vi "Calculate Radius (ball pick up).vi"() -> ()   [LabVIEW 2015]
uses:
  <vilib>/express/express arith-compare/Formula/XNode/ExpressFormulaBlockNode.xnode
panel:
  out "x = y?":bool
  out "Radius 2":dbl
  out "X of intersection":dbl
  out "Radius":dbl
  in  "math tolerance":dbl=0.06
  in  "Ball Y":dbl
  in  "Ball X":dbl
  in  "Min Detect Distance":dbl
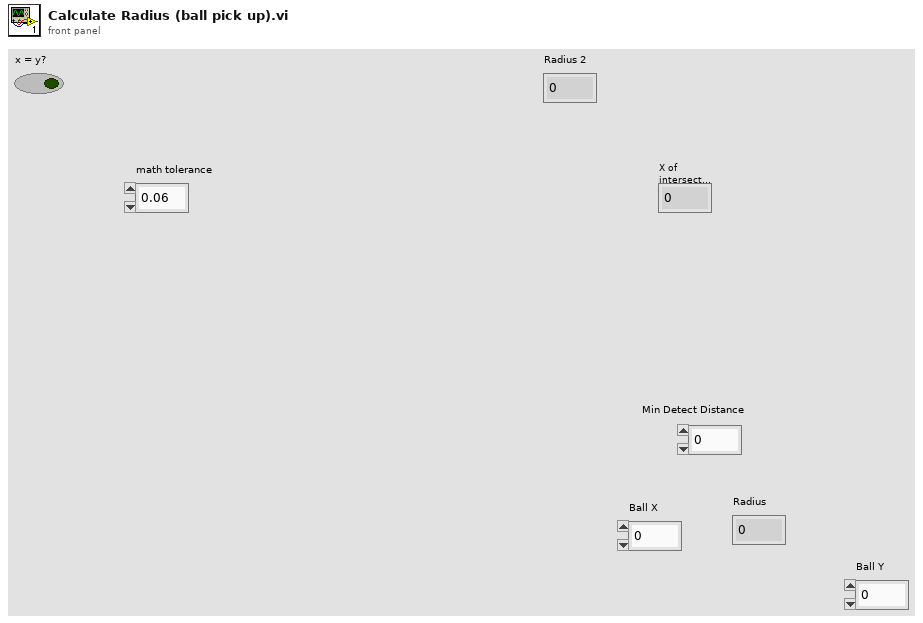
[diagram p1: front panel]
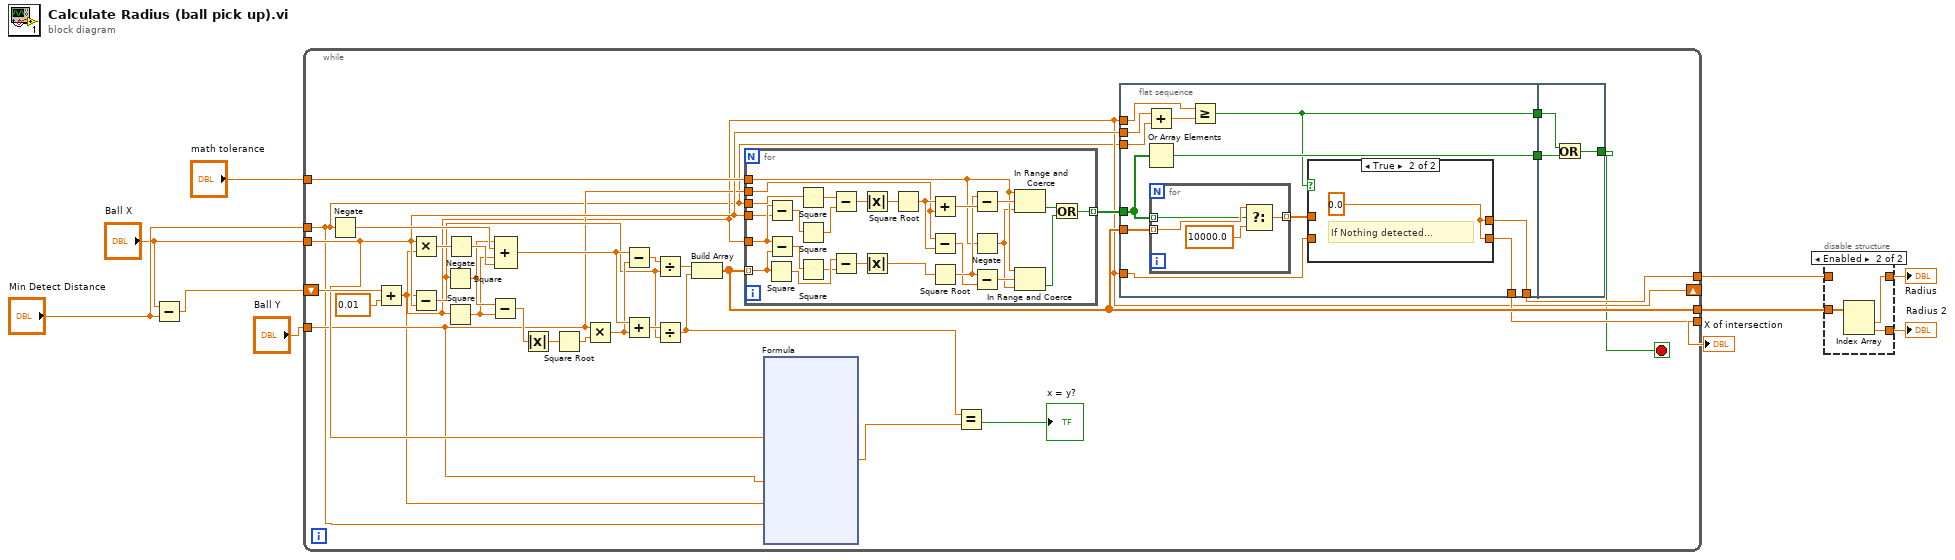
[diagram p0: block diagram]
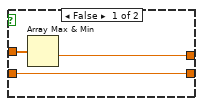
[diagram p3: hidden frame]
diagram:
  n1 = Subtract(x="Ball X", y="Min Detect Distance") -> (x-y=w8:dbl)
  n2 = while {
    tunnel: "Ball X" -> [w18]
    tunnel: "Min Detect Distance" -> [w15]
    shift-right: [w16] -> _
    shift-left: w8 -> [w41]
    tunnel: "Ball Y" -> [w17]
    tunnel: "math tolerance" -> [w26]
    tunnel: [w24] -> w3
    tunnel: [w19] -> w5
    tunnel: [w20] -> w2
    stop <- w11 stop-if-true
    n3 = Negate(x=w15) -> (-x=w39:dbl)
    n4 = Add(x=w41, y=0.01) -> (x+y=w16:dbl)
    n5 = Multiply(x=w18, y=w16) -> (x*y=w38:dbl)
    n6 = Subtract(x=w16, y=w18) -> (x-y=w28:dbl)
    n7 = Square(x=w28) -> (x^2=w35:dbl)
    n8 = Square(x=w16) -> (x^2=w34:dbl)
    n9 = Negate(x=w38) -> (-x=w37:dbl)
    n10 = Subtract(x=w35, y=w34) -> (x-y=w33:dbl)
    n11 = Compound Arithmetic op=ADD(w35, w39, w34, w37) -> (w31:dbl)
    n12 = Absolute Value(x=w33) -> (abs(x)=w21:dbl)
    n13 = Square Root(x=w21) -> (sqrt(x)=w36:dbl)
    n14 = Multiply(x=w17, y=w36) -> (x*y=w30:dbl)
    n15 = Subtract(x=w31, y=w30) -> (x-y=w29:dbl)
    n16 = Add(x=w31, y=w30) -> (x+y=w32:dbl)
    n17 = Divide(x=w29, y=w28) -> (x/y=w27:dbl)
    n18 = Divide(x=w32, y=w28) -> (x/y=w13:dbl)
    n19 = Build Array(w27, w13) -> (w20:dbl[])
    n20 = for {
      tunnel: w20 -> [w103] mode=indexing
      tunnel: w16 -> [w94]
      tunnel: w15 -> [w95]
      tunnel: w18 -> [w93]
      tunnel: w17 -> [w91]
      tunnel: w26 -> [w85]
      tunnel: [w81] -> w25 mode=indexing
      n21 = Square(x=w103) -> (x^2=w104:dbl)
      n22 = Subtract(x=w94, y=w93) -> (x-y=w98:dbl)
      n23 = Subtract(x=w94, y=w103) -> (x-y=w102:dbl)
      n24 = Square(x=w95) -> (x^2=w99:dbl)
      n25 = Square(x=w98) -> (x^2=w97:dbl)
      n26 = Square(x=w102) -> (x^2=w101:dbl)
      n27 = Subtract(x=w99, y=w97) -> (x-y=w96:dbl)
      n28 = Subtract(x=w104, y=w101) -> (x-y=w100:dbl)
      n29 = Absolute Value(x=w96) -> (abs(x)=w80:dbl)
      n30 = Absolute Value(x=w100) -> (abs(x)=w79:dbl)
      n31 = Square Root(x=w80) -> (sqrt(x)=w92:dbl)
      n32 = Add(x=w92, y=w91) -> (x+y=w90:dbl)
      n33 = Subtract(x=w91, y=w92) -> (x-y=w88:dbl)
      n34 = Square Root(x=w79) -> (sqrt(x)=w89:dbl)
      n35 = Subtract(x=w89, y=w90) -> (x-y=w87:dbl)
      n36 = Negate(x=w85) -> (-x=w84:dbl)
      n37 = Subtract(x=w89, y=w88) -> (x-y=w86:dbl)
      n38 = In Range and Coerce(upper limit=w85, x=w87, lower limit=w84) -> (In Range?=w83:bool)  [unwired: 1 out]
      n39 = In Range and Coerce(upper limit=w85, x=w86, lower limit=w84) -> (In Range?=w82:bool)  [unwired: 1 out]
      n40 = Or(x=w83, y=w82) -> (x .or. y?=w81:bool)
    }
    n41 = xnode "Formula"("A"=w18, "B"=w17, "X"=w16, "R1"=w15) -> ("Result"=w14:dbl)  [unwired: 1 in, 1 out]
    n42 = Equal?(x=w13, y=w14) -> (x = y?=→"x = y?":bool)
    n43 = flat-sequence {
      tunnel: w25 -> [w66]
      tunnel: w20 -> [w67]
      tunnel: [w64] -> w24
      tunnel: [w57] -> w23
      tunnel: [w56] -> w22
      tunnel: w16 -> [w63]
      tunnel: w18 -> [w61]
      tunnel: w15 -> [w60]
      tunnel: [w59] -> w19
      tunnel: w16 -> [w58]
      tunnel: [w76] -> w11
      tunnel: w23 -> [w78]
      tunnel: w22 -> [w77]
      frame #0 {
        n44 = Add(x=w61, y=w60) -> (x+y=w62:dbl)
        n45 = Or Array Elements(Boolean array=w66) -> (logical OR=w57:bool)
        n46 = for {
          tunnel: w67 -> [w75] mode=indexing
          tunnel: w66 -> [w74] mode=indexing
          tunnel: [w72] -> w65 mode=indexing
          n47 = Select(t=w75, s=w74, f=10000.0) -> (s? t:f=w72:dbl)
        }
        n48 = Greater Or Equal?(x=w63, y=w62) -> (x >= y?=w56:bool)
        n49 = case shown="True" w56 {
          tunnel: w65 -> [w70 _]
          tunnel: [w69 w71] -> w64
          tunnel: [w68 w71] -> w59
          tunnel: w58 -> [w68 _]
          frame False {
            n50 = Array Max & Min(array=w70) -> (min value=w69:dbl)  [unwired: 3 out]
          }
          frame True {
            w71 = 0.0
            # "If Nothing detected..."
          }
        }
      }
      frame #1 {
        n51 = Or(x=w77, y=w78) -> (x .or. y?=w76:bool)
      }
    }
  }
  "X of intersection" <- w5
  n52 = disable-structure shown="Enabled" {
    disable-tunnel: [w105 w107] -> w4
    disable-tunnel: w3 -> [w105 _]
    disable-tunnel: w2 -> [_ w108]
    disable-tunnel: [_ w106] -> w1
    frame Disabled {
    }
    frame Enabled {
      n53 = Index Array(array=w108) -> (element #1=w107:dbl, element #2=w106:dbl)  [unwired: 2 in]
    }
  }
  "Radius" <- w4
  "Radius 2" <- w1
